vi "Change SP.vi"(1 "error in":errorcluster, 2 "Set Point":u32, 3 "Adress":u8 format="%x", 4 "VISA resource name":refnum<visa-resource-name>="ASRL2::INSTR") -> (0 "error out":errorcluster)   [LabVIEW 2009]
uses:
  <vilib>/Instr/_visa.llb/VISA Configure Serial Port (Instr).vi
panel:
  out "Write buffer":string
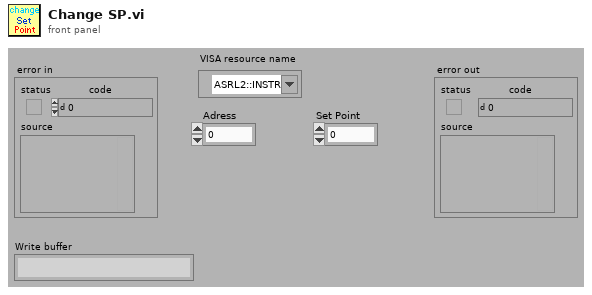
[diagram p1: front panel]
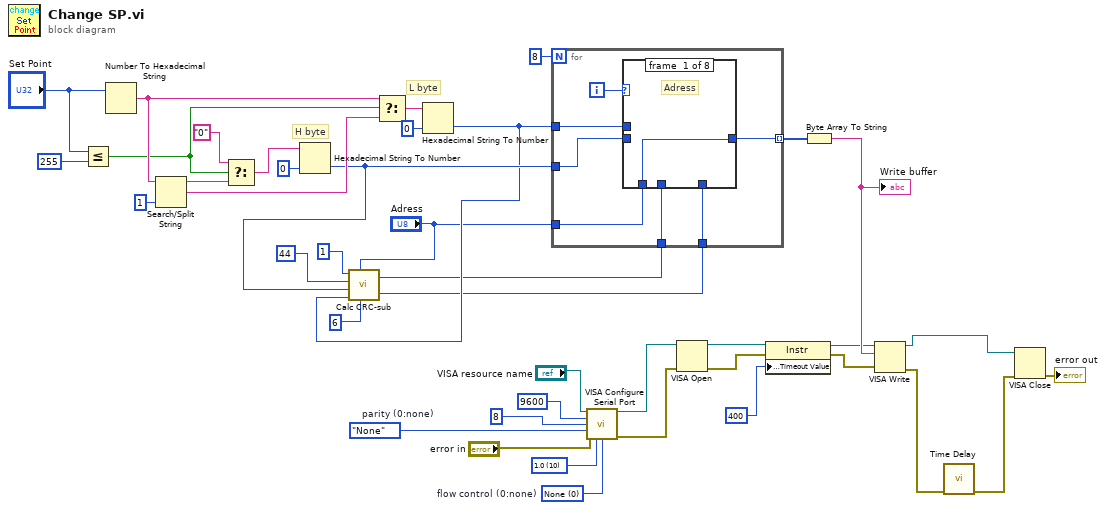
[diagram p0: block diagram]
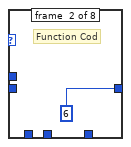
[diagram p2: hidden frame]
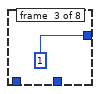
[diagram p3: hidden frame]
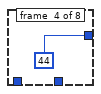
[diagram p4: hidden frame]
diagram:
  w11 = enum16{"None", "Odd", "Even", "Mark", "Space"}."None"  # parity (0:none)
  w7 = u16 0 items=["None"=0, "XON/XOFF"=1, "RTS/CTS"=2, "DTR/DSR"=4]  # flow control (0:none)
  w8 = u16 10 items=["1.0"=10, "1.5"=15, "2.0"=20] ("stop bits (10: 1 bit)")
  # "L byte"
  # "H byte"
  n1 = Less Or Equal?(x="Set Point", y=u32 255) -> (x <= y?=w24:bool)
  n2 = Number To Hexadecimal String(2:"Set Point") -> (0:w30:string)  [unwired: 1 out]
  n3 = Search/Split String(string=w30, offset (0)=1) -> (substring before match=w29:string, match + rest of string=w27:string)  [unwired: 2 out]
  n4 = Select(t="0", s=w24, f=w29) -> (s? t:f=w25:string)
  n5 = Hexadecimal String To Number(string=w25, default (0uL)=u8 0 ("default (0 U32)")) -> (number=w19:u8)  [unwired: 2 out]
  n6 = Select(t=w30, s=w24, f=w27) -> (s? t:f=w26:string)
  n7 = Hexadecimal String To Number(string=w26, default (0uL)=u8 0 ("default (0 U32)")) -> (number=w18:u8)  [unwired: 2 out]
  n8 = call "Calc CRC-sub.vi"("Command"=u8 6, "Adress"="Adress", "Data L"=w18, "Data H"=w19, "Reg L"=u8 44 ("Reg-L"), "Reg H"=u8 1 ("Reg-H")) -> ("L byte"=w17:u8, "H byte"=w16:u8)
  n9 = for {
    N: 8 -> [_]
    tunnel: [w47] -> w41 mode=indexing
    tunnel: w19 -> [w46]
    tunnel: w18 -> [w45]
    tunnel: w17 -> [w44]
    tunnel: w16 -> [w43]
    tunnel: "Adress" -> [w42]
    i -> [w48]
    n10 = case shown="7" w48 {
      tunnel: [w49 u8 6 ("Command") u8 1 ("Reg-H") u8 44 ("Reg-L") w53 w54 w55 w56] -> w47
      tunnel: w46 -> [_ _ _ _ w53 _ _ _]
      tunnel: w45 -> [_ _ _ _ _ w54 _ _]
      tunnel: w44 -> [_ _ _ _ _ _ w55 _]
      tunnel: w43 -> [_ _ _ _ _ _ _ w56]
      tunnel: w42 -> [w49 _ _ _ _ _ _ _]
      frame #0 {
        # "Adress"
      }
      frame #1 {
        # "Function Cod"
      }
      frame #2 {
      }
      frame #3 {
      }
      frame #4 {
        # "Data H"
      }
      frame #5 {
        # "Data L"
      }
      frame #6 {
        # "CRC-L"
      }
      frame #7 {
        # "CRC-H"
      }
    }
  }
  n11 = call-poly "VISA Configure Serial Port"("VISA resource name"="VISA resource name", "baud rate (9600)"=u32 9600, "data bits (8)"=u16 8, "parity (0:none)"=w11, "error in (no error)"="error in", "stop bits (10: 1 bit)"=w8, "flow control (0:none)"=w7) -> ("VISA resource name out"=w4:refnum<visa-resource-name>, "error out"=w3:errorcluster)  [unwired: 7 out]
  n12 = VISA Open(error in (no error)=w3, VISA resource name=w4) -> (VISA resource name=w36:refnum<visa-resource-name>, error out=w35:errorcluster)  [unwired: 3 out]
  n13 = property class="Instr"(reference=w36, error in=w35, "General Settings:Timeout Value"=u32 400) -> (reference out=w34:refnum<visa-resource-name>, error out=w33:errorcluster)
  n14 = Byte Array To String(unsigned byte array=w41) -> (string=w38:string)
  "Write buffer" <- w38
  n15 = VISA Write(VISA resource name=w34, write buffer=w38, error in (no error)=w33) -> (VISA resource name out=w1:refnum<visa-resource-name>, error out=w12:errorcluster)  [unwired: 1 out]
  n16 = call "Time Delay"("error in (no error)"=w12) -> ("error out"=w2:errorcluster)  [unwired: 1 in, 9 out]
  n17 = VISA Close(VISA resource name=w1, error in (no error)=w2) -> (error out=→"error out":errorcluster)
